vi "Robot Global Data.vi"() -> ()   [LabVIEW 2011]
doc: "This global VI can contain as many global variables as you need. Place a control on the panel, give it a good name. To read or write to it from a VI, drag the icon to the diagram of that VI. You can also drag from the project. Click on the node to change which global you access. You shouldn't have multiple locations writing to a global or it will cause a race-condition."
uses:
  <vilib>/Rock Robotics/WPI/Camera/WPI_CameraImageSize.ctl
panel:
  out "WhereAmIString?":string
  in  "WhereAmI":T1(ring)
  in  "State":T2(ring)
  in  "ShooterControl":bool
  in  "FullSpeedShooter":bool
  out "DriverControl":bool
  out "InRange?":bool
  in  "Kicker Restored?":bool
  in  "Collector?":bool
  in  "3Ball'sIn":bool
  out "UltrasonicDistance":dbl
  in  "CurentSpeed":dbl
  in  "ShooterSpeedWanted":dbl
  in  "Sensitive":bool
  out "Reset":bool
  in  "BridgeUp":bool
  out "BridgeDown":dbl
  out "Kicker":bool
  out "LeftRobotDrive":dbl
  out "RightRobotDrive":dbl
  out "Accelerator":dbl
  out "Collector":dbl
  in  "LED toggle rate (ms)":u32=20
  in  "image size":T3=enum."320x240"
  in  "Enable Vision":bool
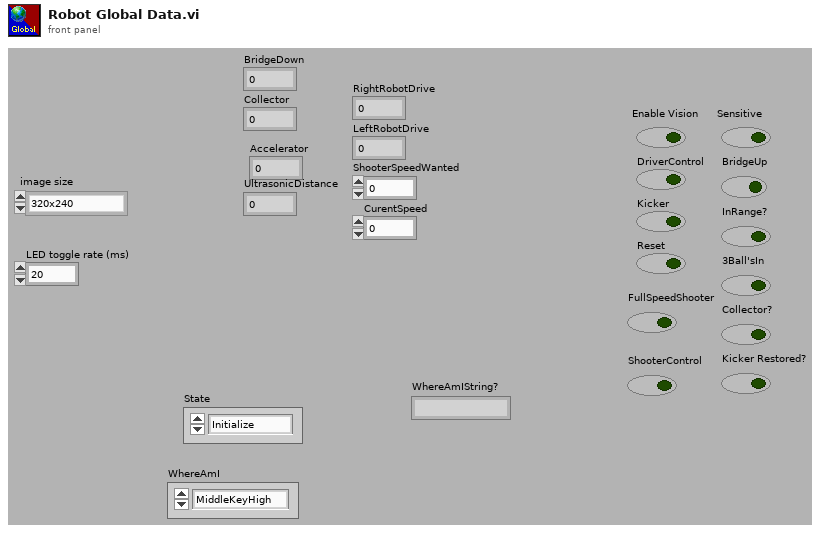
[diagram p1: front panel]
types:
  T1 = enum16{"MiddleKeyHigh", "MiddleKeyLow", "SidesKey"}
  T2 = enum16{"Initialize", "Delay", "Drive", "GetSpeed", "Shoot", "Spin", "DriveToBridge", "Finish"}
  T3 = typedef "WPI_CameraImageSize.ctl" = enum16{"640x480", "320x240", "160x120"}
diagram:
